vi "VoltageMeanRead.vi"(8 "error in":errorcluster, 11 "refnum":refnum<file>) -> (0 "error out":errorcluster, 3 "refnum out":refnum<file>)   [LabVIEW 2009]
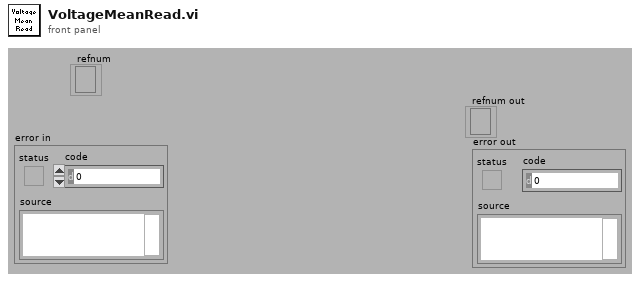
[diagram p1: front panel]
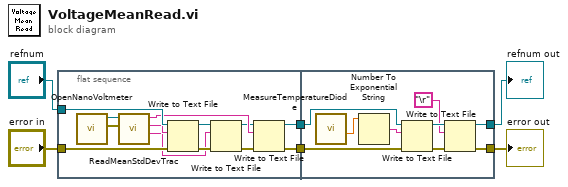
[diagram p0: block diagram]
diagram:
  n1 = flat-sequence {
    tunnel: "refnum" -> [w19]
    tunnel: "error in" -> [w18]
    tunnel: [w12] -> w6
    tunnel: [w7] -> w1
    tunnel: [w23] -> w3
    tunnel: [w22] -> w2
    tunnel: w6 -> [w21]
    tunnel: w1 -> [w20]
    frame #0 {
      n2 = call "OpenNanoVoltmeter.vi"() -> ("error out"=w17:errorcluster, "reference out"=w16:refnum<visa-resource-name>)  [unwired: 8 in]
      n3 = call "ReadMeanStdDevTrac.vi"("error in"=w17, "reference in 3"=w16) -> ("STDDEV"=w11:string, "MEAN"=w15:string, "TRACEr"=w10:string)  [unwired: 5 in, 2 out]
      n4 = Write to Text File(file (use dialog)=w19, text=w15, error in=w18) -> (refnum out=w9:refnum<file>, error out=w14:errorcluster)  [unwired: 1 in, 1 out]
      n5 = Write to Text File(file (use dialog)=w9, text=w11, error in=w14) -> (refnum out=w8:refnum<file>, error out=w13:errorcluster)  [unwired: 1 in, 1 out]
      n6 = Write to Text File(file (use dialog)=w8, text=w10, error in=w13) -> (refnum out=w7:refnum<file>, error out=w12:errorcluster)  [unwired: 1 in, 1 out]
    }
    frame #1 {
      n7 = call "MeasureTemperatureDiode.vi"() -> ("Celcius"=w25:dbl)  [unwired: 8 in, 3 out]
      n8 = Number To Exponential String(number=w25) -> (E-format string=w28:string)  [unwired: 3 in]
      n9 = Write to Text File(file (use dialog)=w20, text=w28, error in=w21) -> (refnum out=w26:refnum<file>, error out=w27:errorcluster)  [unwired: 1 in, 1 out]
      n10 = Write to Text File(file (use dialog)=w26, text="\r", error in=w27) -> (refnum out=w23:refnum<file>, error out=w22:errorcluster)  [unwired: 1 in, 1 out]
    }
  }
  "refnum out" <- w3
  "error out" <- w2
